vi "StartSync.vi"(8 "error in (no error)":errorcluster, 11 "NiPxi6682":refnum<class "NiPxi6682.lvclass">) -> (0 "error out":errorcluster, 3 "NiPxi6682":refnum<class "NiPxi6682.lvclass">)   [LabVIEW 2014, in "SyncPlugins.lvlib" / "NiPxi6682.lvclass"]
uses:
  NiPxi6682.lvclass
  NiPxi6682.lvclass/NiPxi6682.ctl
  SyncPluginBase/SyncPluginBase.lvclass/SyncPluginBase.ctl
  Accessors/Read PgmPPSFreq.vi
  Accessors/Read PgmPPS.vi
  Accessors/Read 1PPS.vi
  Accessors/Read NiSyncHandle.vi
  SyncPluginBase/Accessors/Write Run.vi
  SyncPluginBase/Accessors/Write Initiated.vi
  Accessors/Write NiSyncHandle.vi
  <instrlib>/niSync/niSync.llb/niSync Create Clock (Frequency).vi
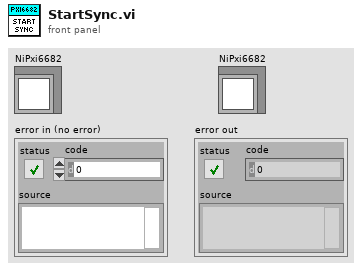
[diagram p1: front panel]
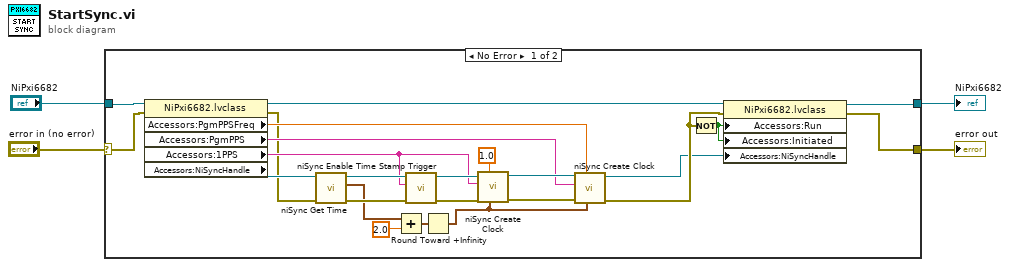
[diagram p0: block diagram]
diagram:
  n1 = case shown="No Error" "error in (no error)" {
    selector: "error in (no error)" -> [w7 w29]
    tunnel: "NiPxi6682" -> [w8 w30]
    tunnel: [w28 w30] -> w2
    tunnel: [w27 w29] -> w1
    frame No Error {
      n2 = property class="NiPxi6682.lvclass"(reference=w8, error in=w7) -> (reference out=w16:refnum<class "NiPxi6682.lvclass">, error out=w17:errorcluster, "Accessors:PgmPPSFreq"=w21:dbl, "Accessors:PgmPPS"=w19:tag, "Accessors:1PPS"=w18:tag, "Accessors:NiSyncHandle"=w26:refnum<k15>)
      n3 = call <instrlib>:"niSync Get Time.vi"("error in (no error)"=w17, "instrument handle"=w26) -> ("error out"=w15:errorcluster, "time"=w12:timestamp, "instrument handle out"=w25:refnum<k15>)  [unwired: 5 in]
      n4 = Add(x=w12, y=2.0) -> (x+y=w10:timestamp)
      n5 = call <instrlib>:"niSync Enable Time Stamp Trigger.vi"("error in (no error)"=w15, "terminal"=w18, "instrument handle"=w25) -> ("error out"=w14:errorcluster, "instrument handle out"=w24:refnum<k15>)  [unwired: 6 in]
      n6 = Round Toward +Infinity(x=w10) -> (ceil(x): smallest int >= x=w9:timestamp)
      n7 = call-poly <instrlib>:"niSync Create Clock.vi"("start time"=w9, "frequency"=1.0, "error in (no error)"=w14, "terminal"=w18, "instrument handle"=w24) -> ("error out"=w13:errorcluster, "instrument handle out"=w23:refnum<k15>)  [unwired: 3 in, 2 out]
      n8 = call-poly <instrlib>:"niSync Create Clock.vi"("start time"=w9, "frequency"=w21, "error in (no error)"=w13, "terminal"=w19, "instrument handle"=w23) -> ("error out"=w22:errorcluster, "instrument handle out"=w6:refnum<k15>)  [unwired: 3 in, 2 out]
      n9 = Not(x=w22) -> (.not. x?=w5:bool)
      n10 = property class="NiPxi6682.lvclass"(reference=w16, error in=w22, "Accessors:Run"=w5, "Accessors:Initiated"=w5, "Accessors:NiSyncHandle"=w6) -> (reference out=w28:refnum<class "NiPxi6682.lvclass">, error out=w27:errorcluster)
    }
    frame Error {
    }
  }
  "NiPxi6682" <- w2
  "error out" <- w1
